vi "raggio_medio(SubVI).vi"(8 "error in (no error)":errorcluster, 11 "Radial Points":cluster{"X":sgl, "Y":sgl}[](array[cluster]) {"Y" format="%.2f"; "X" format="%.2f"}) -> (0 "error out":errorcluster, 3 "Radius":dbl)   [LabVIEW 2020]
uses:
  <vilib>/vision/NI_Vision_Development_Module.lvlib
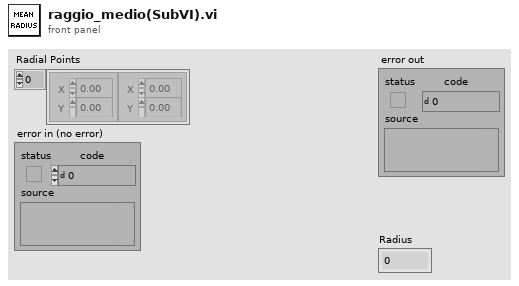
[diagram p1: front panel]
types:
  T1 = cluster{"Center":cluster{"X":sgl, "Y":sgl}, "Radius":dbl}
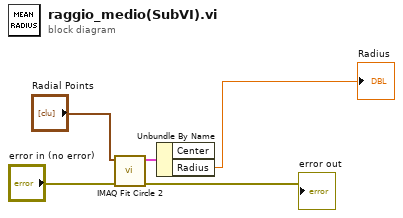
[diagram p0: block diagram]
diagram:
  n1 = call "IMAQ Fit Circle 2"("error in (no error)"="error in (no error)", "Radial Points"="Radial Points") -> ("error out"=→"error out":errorcluster, "Circle"=w5:T1)  [unwired: 4 in, 4 out]
  n2 = Unbundle By Name(w5) -> ("Radius"=→"Radius":dbl)  [unwired: 1 out]
